vi "convertDATACluster.vi"(0 "Variable header":string[](array[string]), 5 "Alias":string[](array[string]), 7 "Array 6":bool[](array[boolean]), 9 "Data in":string[][](array[string]), 12 "variant in":variant) -> (2 "Array of VData":variant[](array[variant]), 3 "type":T5[](array[typedef]) format="%.0x", 4 "Array 2":u32[](array[numeric]), 6 "userID":string, 8 "Array":T5[](array[typedef]) format="%.0x", 10 "Array 3":u32[](array[numeric]), 13 "post time":u32, 14 "Array 4":u32[](array[numeric]), 15 "variant out":variant)   [LabVIEW 2011]
uses:
  <userlib>/_OpenG.lib/lvdata/lvdata.llb/Type Descriptor Enumeration__ogtk.ctl
  dataTypdef.ctl
  <vilib>/vision/Image Controls.llb/IMAQ Image.ctl
  ROIStartfromCam_typdef.ctl
  classicROI_typDef.ctl
  <userlib>/_OpenG.lib/array/array.llb/Sort 2D Array (I32)__ogtk.vi
  <vilib>/vision/NI_Vision_Development_Module.lvlib
panel:
  out "element Name":string[](array[string])
  out "index Array":i32[][](array[numeric])
  out "Sorted Array out":i32[][](array[numeric])
  out "clusterIndex (stop)":i32[](array[numeric])
  out "Array 5":variant[](array[variant])
  out "clusterIndex":i32[](array[numeric])
  out "Cluster Names":string[](array[string])
  out "data 3":T1
  in  "Cam2":T1
  out "VCluster 2":variant
  out "deleted portion":variant[](array[variant])
  out "Array 9":variant[](array[variant])
  out "VCluster":variant
  out "Names (Array)":string[](array[string])
  out "Array 8":bool[](array[boolean])
  out "Array 7":i32[](array[numeric])
  out "data 2":T2
  in  "data":T2
  out "transposed array":string[][](array[string])
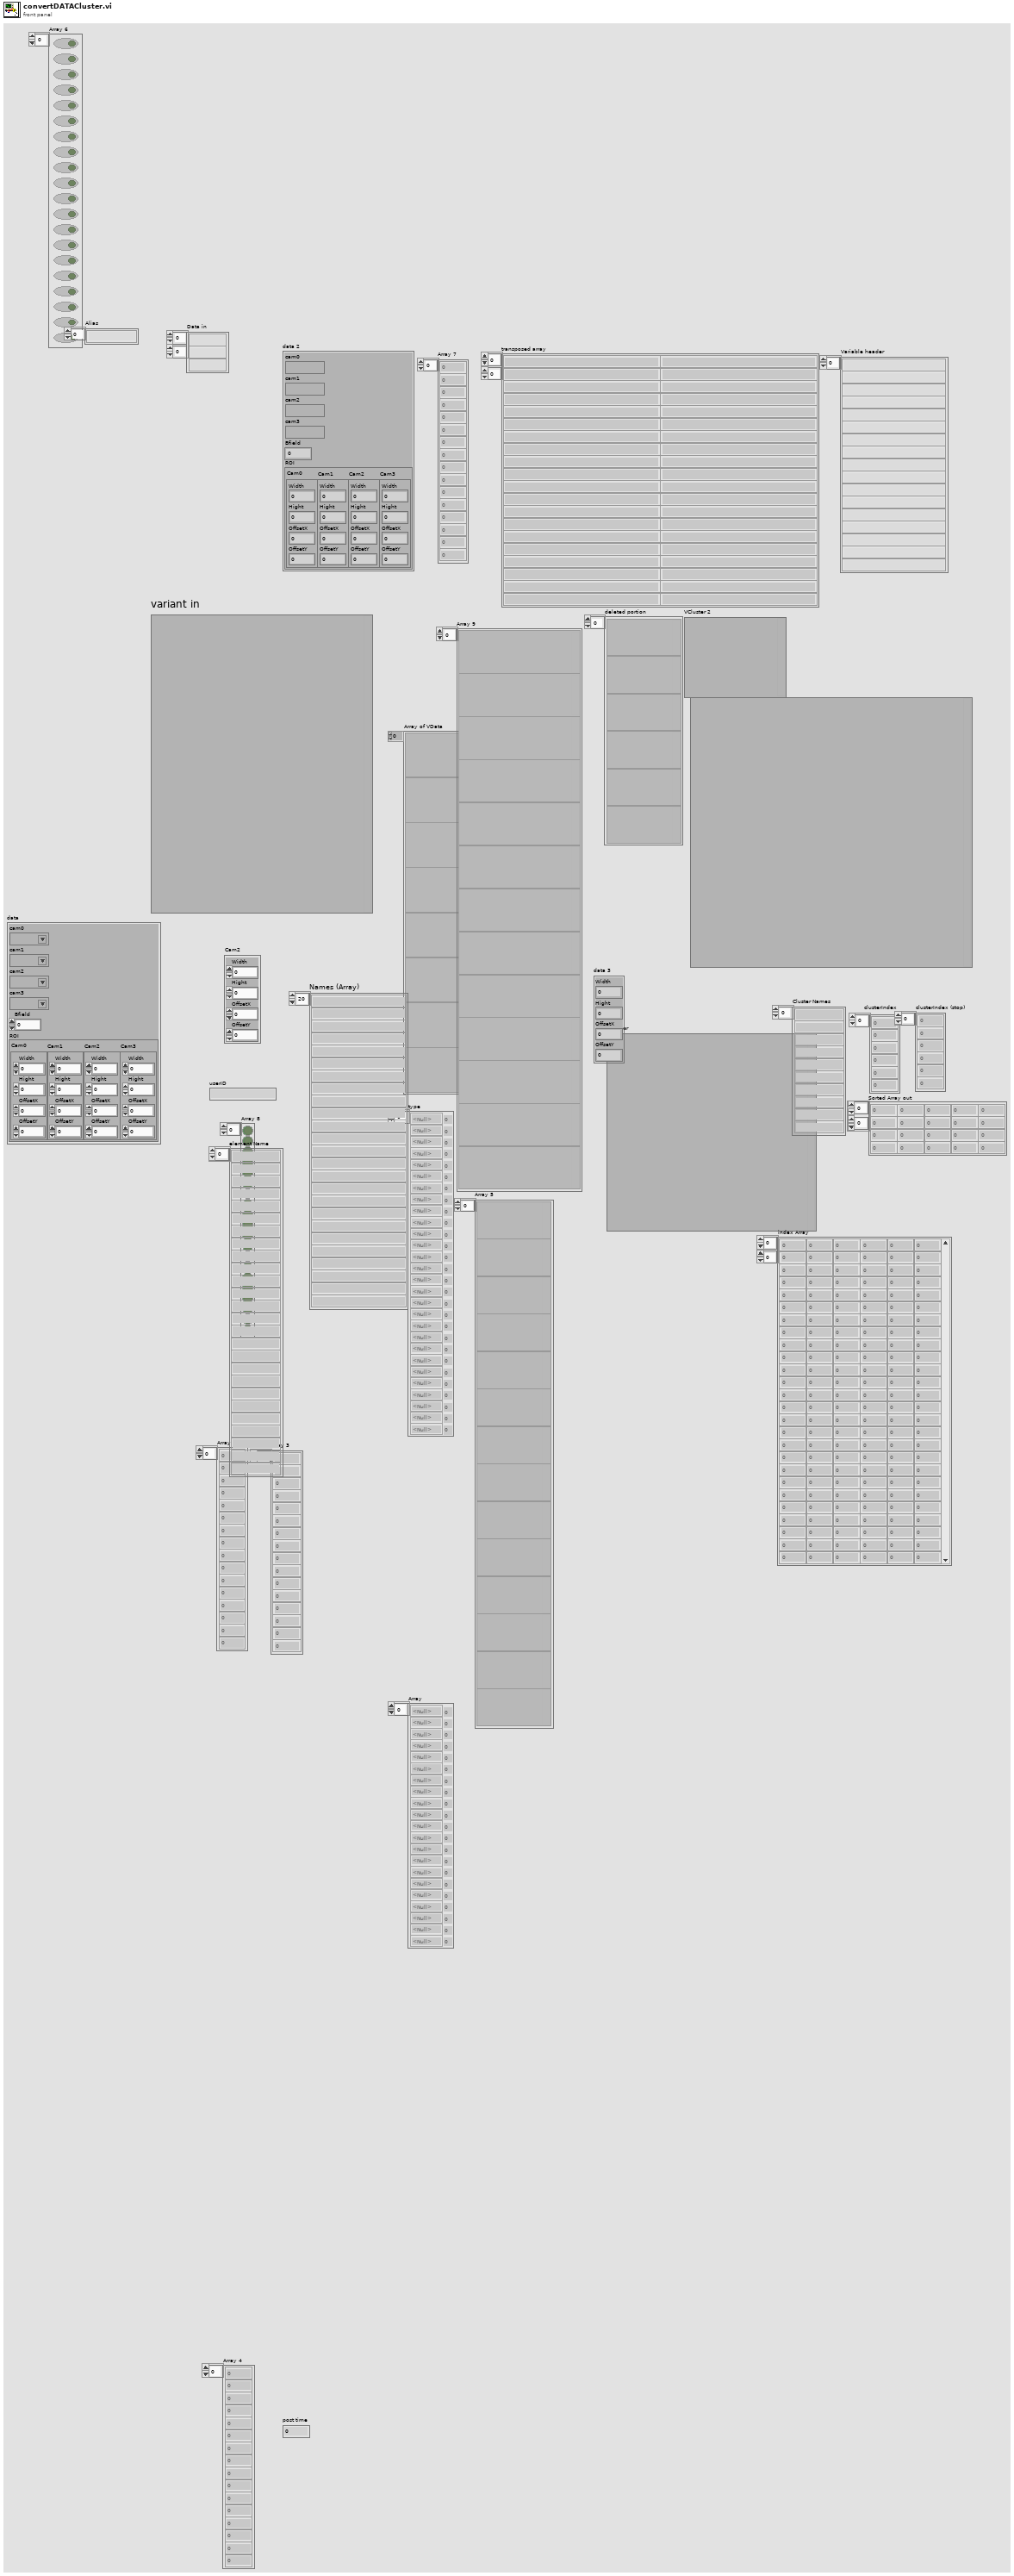
[diagram p1: front panel]
types:
  T1 = typedef "classicROI_typDef.ctl" = cluster{"Width":dbl, "Hight":dbl, "OffsetX":dbl, "OffsetY":dbl}
  T2 = typedef "dataTypdef.ctl" = cluster{"cam0":T3, "cam1":T3, "cam2":T3, "cam3":T3, "Bfield":dbl, "ROI":T4}
  T3 = typedef "IMAQ Image.ctl" = refnum<image>
  T4 = typedef "ROIStartfromCam_typdef.ctl" = cluster{"Cam0":T1, "Cam1":T1, "Cam2":T1, "Cam3":T1}
  T5 = typedef "Type Descriptor Enumeration__ogtk.ctl" = enum8{"<Null>", "I8", "I16", "I32", "I64", "U8", "U16", "U32", "U64", "SGL", "DBL", "EXT", "CSG", "CDB", "CXT", "0x0F", "0x10", "0x11", "0x12", "0x13", "0x14", "Enum U8", "Enum U16", "Enum U32", "Enum U64", "SGL PQ", "DBL PQ", "EXT PQ", "CSG PQ", "CDB PQ", "CXT PQ", "0x1F", "0x20", "Boolean", "0x22", "0x23", "0x24", "0x25", "0x26", "0x27", "0x28", "0x29", "0x2A", "0x2B", "0x2C", "0x2D", "0x2E", "0x2F", "String", "0x31", "Path", "Pict", "0x34", "0x35", "0x36", "DAQ", "0x38", "0x39", "0x3A", "0x3B", "0x3C", "0x3D", "0x3E", "0x3F", "Array", "0x41", "0x42", "0x43", "0x44", "0x45", "0x46", "0x47", "0x48", "0x49", "0x4A", "0x4B", "0x4C", "0x4D", "0x4E", "0x4F", "Cluster", "0x51", "0x52", "Variant", "Waveform", "0x55", "0x56", "0x57", "0x58", "0x59", "0x5A", "0x5B", "0x5C", "0x5D", "0x5E", "0x5F", "0x60", "0x61", "0x62", "0x63", "0x64", "0x65", "0x66", "0x67", "0x68", "0x69", "0x6A", "0x6B", "0x6C", "0x6D", "0x6E", "0x6F", "Refnum"}
  T6 = typedef "Image Type" = u32
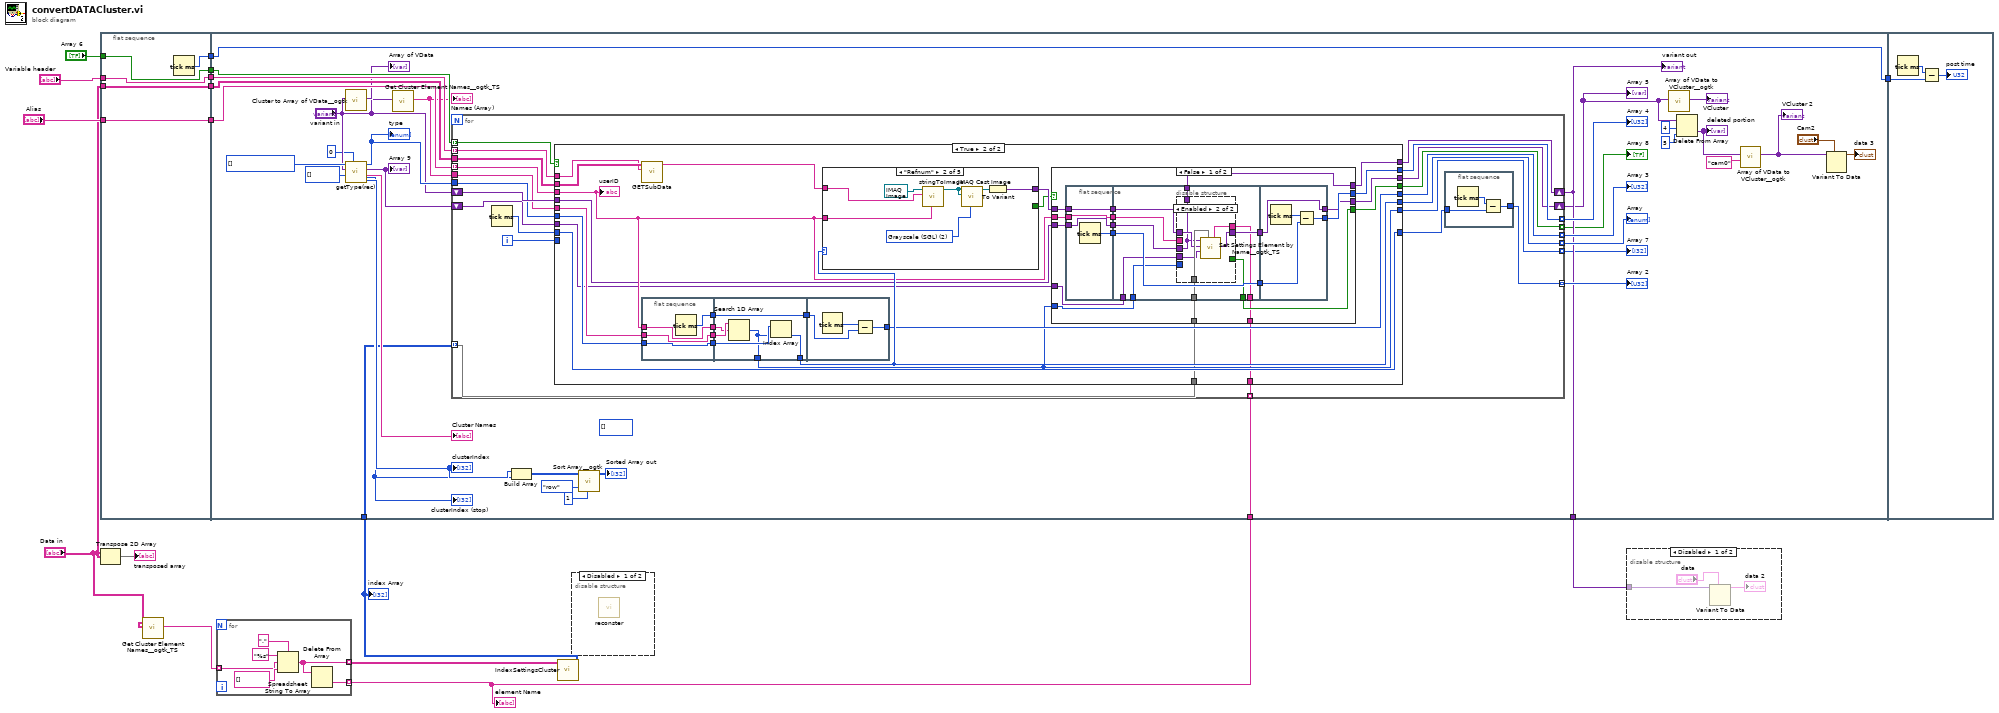
[diagram p0: block diagram]
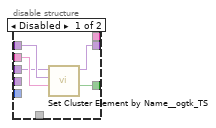
[diagram p5: hidden frame]
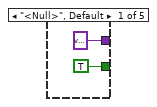
[diagram p7: hidden frame]
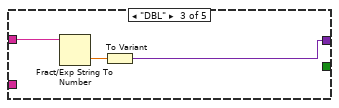
[diagram p8: hidden frame]
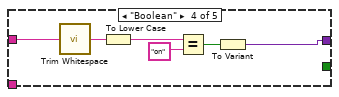
[diagram p9: hidden frame]
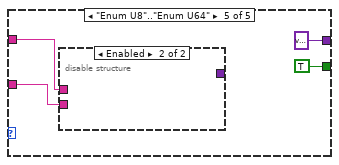
[diagram p10: hidden frame]
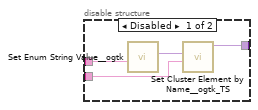
[diagram p11: hidden frame]
diagram:
  n1 = flat-sequence {
    tunnel: "Array 6" -> [w18]
    tunnel: "Alias" -> [w19]
    tunnel: "Data in" -> [w20]
    tunnel: "Variable header" -> [w21]
    tunnel: [w21] -> w16
    tunnel: [w20] -> w15
    tunnel: [w19] -> w14
    tunnel: [w18] -> w13
    tunnel: [w17] -> w12
    tunnel: w16 -> [w59]
    tunnel: w15 -> [w58]
    tunnel: w14 -> [w51]
    tunnel: w13 -> [w57]
    tunnel: w12 -> [w56]
    tunnel: [w56] -> w11
    tunnel: [w45] -> w6
    tunnel: w4 -> [w23]
    tunnel: w1 -> [w22]
    tunnel: w11 -> [w201]
    frame #0 {
      n2 = Tick Count (ms)() -> (millisecond timer value=w17:u32)
    }
    frame #1 {
      (unwired) i32[] [] ("clusterinex")
      w52 = T5[] [] items=["<Null>", "I8", "I16", "I32", "I64", "U8", "U16", "U32", "U64", "SGL", "DBL", "EXT", "CSG", "CDB", "CXT", "0x0F", "0x10", "0x11", "0x12", "0x13", "0x14", "Enum U8", "Enum U16", "Enum U32", "Enum U64", "SGL PQ", "DBL PQ", "EXT PQ", "CSG PQ", "CDB PQ", "CXT PQ", "0x1F", "0x20", "Boolean", "0x22", "0x23", "0x24", "0x25", "0x26", "0x27", "0x28", "0x29", "0x2A", "0x2B", "0x2C", "0x2D", "0x2E", "0x2F", "String", "0x31", "Path", "Pict", "0x34", "0x35", "0x36", "DAQ", "0x38", "0x39", "0x3A", "0x3B", "0x3C", "0x3D", "0x3E", "0x3F", "Array", "0x41", "0x42", "0x43", "0x44", "0x45", "0x46", "0x47", "0x48", "0x49", "0x4A", "0x4B", "0x4C", "0x4D", "0x4E", "0x4F", "Cluster", "0x51", "0x52", "Variant", "Waveform", "0x55", "0x56", "0x57", "0x58", "0x59", "0x5A", "0x5B", "0x5C", "0x5D", "0x5E", "0x5F", "0x60", "0x61", "0x62", "0x63", "0x64", "0x65", "0x66", "0x67", "0x68", "0x69", "0x6A", "0x6B", "0x6C", "0x6D", "0x6E", "0x6F", "Refnum"] ("type in")
      n3 = call <userlib>:"Cluster to Array of VData__ogtk.vi"("Cluster"="variant in") -> ("Array of VData"=→"Array of VData":variant[])  [unwired: 9 in, 1 out]
      n4 = call "getType(rec).vi"("index"=0, "clusterIndex (start)"=i32[] [], "variant in"="variant in", "type in"=w52) -> ("clusterIndex (start)"=w29:i32[], "Cluster Names"=→"Cluster Names":string[], "Array 2"=w42:variant[], "Array"=w49:T5[], "clusterIndex (stop)"=w28:i32[])  [unwired: 2 in, 1 out]
      "type" <- w49
      "Array 9" <- w42
      "clusterIndex" <- w29
      "clusterIndex (stop)" <- w28
      n5 = call "Get Cluster Element Names__ogtk_TS.vi"("Variant"="variant in") -> ("Names (Array)"=w47:string[])  [unwired: 9 in, 1 out]
      "Names (Array)" <- w47
      n6 = for {
        tunnel: w58 -> [w79]
        shift-right: [w80] -> w45
        shift-left: "variant in" -> [w77]
        tunnel: w59 -> [w78] mode=indexing
        tunnel: w51 -> [w76] mode=indexing
        tunnel: w57 -> [w75] mode=indexing
        tunnel: [w74] -> w55 mode=indexing
        tunnel: [w71] -> w54 mode=indexing
        tunnel: [w70] -> w53 mode=indexing
        tunnel: w49 -> [w68]
        tunnel: w47 -> [w67]
        tunnel: [w66] -> w46 mode=indexing
        tunnel: [w65] -> w44 mode=indexing
        tunnel: [w64] -> w43 mode=indexing
        shift-right: [w62] -> w31
        shift-left: w42 -> [w63]
        tunnel: w23 -> [w61] mode=indexing
        tunnel: w22 -> [w60] mode=indexing
        i -> [w69]
        n7 = Tick Count (ms)() -> (millisecond timer value=w73:u32)
        n8 = case shown="True" w75 {
          tunnel: [w86 w98] -> w80
          tunnel: w79 -> [_ w111]
          tunnel: w78 -> [_ w110]
          tunnel: w77 -> [w86 w92]
          tunnel: w76 -> [_ w96]
          tunnel: [_ w105] -> w74
          tunnel: w73 -> [w85 w108]
          tunnel: [w85 w108] -> w72
          tunnel: [_ w99] -> w70
          tunnel: w69 -> [_ _]
          tunnel: w68 -> [_ w106]
          tunnel: w67 -> [_ w107]
          tunnel: [_ w94] -> w66
          tunnel: [_ w89] -> w65
          tunnel: [_ w93] -> w64
          tunnel: w63 -> [w84 w91]
          tunnel: [w84 w90] -> w62
          tunnel: w61 -> [_ w88]
          tunnel: w60 -> [_ w87]
          frame False {
          }
          frame True {
            n9 = call "GETSubData.vi"("Variable Header"=w110, "Data out"=w111) -> ("delimiter (Tab)"=w109:string)  [unwired: 9 in]
            n10 = flat-sequence {
              tunnel: w106 -> [w162]
              tunnel: w96 -> [w163]
              tunnel: w107 -> [w164]
              tunnel: [w164] -> w104
              tunnel: [w163] -> w103
              tunnel: [w162] -> w102
              tunnel: [w161] -> w101
              tunnel: [w167] -> w105
              tunnel: w104 -> [w170]
              tunnel: w103 -> [w169]
              tunnel: w102 -> [w168]
              tunnel: w101 -> [w166]
              tunnel: [w166] -> w100
              tunnel: [w165] -> w89
              tunnel: w100 -> [w172]
              tunnel: [w171] -> w99
              frame #0 {
                n11 = Tick Count (ms)() -> (millisecond timer value=w161:u32)
              }
              frame #1 {
                n12 = Search 1D Array(1D array=w170, element=w169) -> (index of element=w165:i32)  [unwired: 1 in]
                n13 = Index Array(array=w168, index=w165) -> (element=w167:T5)
              }
              frame #2 {
                n14 = Tick Count (ms)() -> (millisecond timer value=w173:u32)
                n15 = Subtract(x=w173, y=w172) -> (x-y=w171:u32)
              }
            }
            n16 = case shown="\"Refnum\"" w105 {
              tunnel: w109 -> [_ w182 w185 w191 w195]
              tunnel: w96 -> [_ w176 _ _ w194]
              tunnel: [variant ("Variant") w177 w183 w186 variant ("Variant")] -> w97
              tunnel: [TRUE _ _ _ TRUE] -> w95
              frame "<Null>", Default {
              }
              frame "Refnum" {
                w180 = T6 2 items=["Grayscale (U8)", "Grayscale (I16)", "Grayscale (SGL)", "Complex (CSG)", "RGB (U32)", "HSL (U32)", "RGB (U64)", "Grayscale (U16)"] ("Image Type")
                n17 = call "stringToImage.vi"("label text (image name)"=w176, "data out"=w182, "Refnum in"=T3 refnum ("Image")) -> ("Refnum out"=w181:T3)  [unwired: 5 in, 3 out]
                n18 = call "IMAQ Cast Image"("Image Type"=w180, "Image Dst"=w181, "Image Src"=w181) -> ("Image Dst Out"=w178:T3)  [unwired: 7 in, 1 out]
                n19 = To Variant(anything=w178) -> (Variant=w177:variant)
              }
              frame "DBL" {
                n20 = Fract/Exp String To Number(string=w185) -> (number=w184:dbl)  [unwired: 3 in, 1 out]
                n21 = To Variant(anything=w184) -> (Variant=w183:variant)
              }
              frame "Boolean" {
                n22 = call <vilib>:"Trim Whitespace.vi"("string"=w191) -> ("trimmed string"=w190:string)  [unwired: 1 in]
                n23 = To Lower Case(string=w190) -> (all lower case string=w189:string)
                n24 = Equal?(x=w189, y="on" ("x")) -> (x = y?=w187:bool)
                n25 = To Variant(anything=w187) -> (Variant=w186:variant)
              }
              frame "Enum U8".."Enum U64" {
                n26 = disable-structure shown="Enabled" {
                  disable-tunnel: w195 -> [w199 _]
                  disable-tunnel: w194 -> [w198 _]
                  disable-tunnel: [w196 _] -> _
                  frame Disabled {
                    n27 = call <userlib>:"Set Enum String Value__ogtk.vi"("String Value"=w199) -> ("Enum"=w197:variant)  [unwired: 9 in, 1 out]
                    n28 = call "Set Cluster Element by Name__ogtk_TS.vi"("Element Name (\"\": New Element Data Name)"=w198, "New Element Value"=w197) -> ("VCluster out"=w196:variant)  [unwired: 7 in, 2 out]
                  }
                  frame Enabled {
                  }
                }
              }
            }
            n29 = case shown="False" w95 {
              tunnel: w92 -> [w128 w160]
              tunnel: [w113 w160] -> w98
              tunnel: w97 -> [w127 _]
              tunnel: w96 -> [w126 _]
              tunnel: [w120 _] -> w94
              tunnel: [w119 _] -> w93
              tunnel: w91 -> [w117 w159]
              tunnel: [w114 w159] -> w90
              tunnel: w89 -> [w116 _]
              tunnel: w88 -> [w115 _]
              tunnel: w87 -> [w112 _]
              frame False {
                n30 = flat-sequence {
                  tunnel: w126 -> [w130]
                  tunnel: w127 -> [w131]
                  tunnel: w128 -> [w132]
                  tunnel: [w132] -> w125
                  tunnel: [w131] -> w124
                  tunnel: [w130] -> w123
                  tunnel: [w129] -> w122
                  tunnel: w125 -> [w138]
                  tunnel: w124 -> [w140]
                  tunnel: w123 -> [w141]
                  tunnel: w122 -> [w143]
                  tunnel: [w143] -> w121
                  tunnel: [w142] -> w119
                  tunnel: [w139] -> w118
                  tunnel: w117 -> [w137]
                  tunnel: w116 -> [w136]
                  tunnel: w115 -> [w135]
                  tunnel: [w134] -> w113
                  tunnel: w112 -> [w133]
                  tunnel: w121 -> [w157]
                  tunnel: [w156] -> w120
                  tunnel: w118 -> [w155]
                  tunnel: [w155] -> w114
                  frame #0 {
                    n31 = Tick Count (ms)() -> (millisecond timer value=w129:u32)
                  }
                  frame #1 {
                    n32 = disable-structure shown="Enabled" {
                      disable-tunnel: [w148 _] -> w142
                      disable-tunnel: w141 -> [w147 _]
                      disable-tunnel: w140 -> [w146 w153]
                      disable-tunnel: [w145 w151] -> w139
                      disable-tunnel: w138 -> [w144 w150]
                      disable-tunnel: w137 -> [_ w152]
                      disable-tunnel: w136 -> [_ _]
                      disable-tunnel: w135 -> [_ w154]
                      disable-tunnel: [_ w150] -> w134
                      disable-tunnel: w133 -> [_ w149]
                      frame Disabled {
                        n33 = call "Set Cluster Element by Name__ogtk_TS.vi"("Element Name (\"\": New Element Data Name)"=w147, "New Element Value"=w146, "Cluster"=w144) -> ("found?"=w148:bool, "VCluster out"=w145:variant)  [unwired: 6 in, 1 out]
                      }
                      frame Enabled {
                        n34 = call "Set Settings Element by Name__ogtk_TS.vi"("element Name"=w149, "index Array"=w154, "Settings VData"=w152, "New Element Value"=w153, "Cluster"=w150) -> ("Settings VData out"=w151:variant[])  [unwired: 5 in, 1 out]
                      }
                    }
                  }
                  frame #2 {
                    n35 = Tick Count (ms)() -> (millisecond timer value=w158:u32)
                    n36 = Subtract(x=w158, y=w157) -> (x-y=w156:u32)
                  }
                }
              }
              frame True {
              }
            }
            "userID" <- w96
          }
        }
        n37 = flat-sequence {
          tunnel: w72 -> [w82]
          tunnel: [w81] -> w71
          frame #0 {
            n38 = Tick Count (ms)() -> (millisecond timer value=w83:u32)
            n39 = Subtract(x=w83, y=w82) -> (x-y=w81:u32)
          }
        }
      }
      "variant out" <- w45
      "Array" <- w55
      "Array 2" <- w54
      "Array 3" <- w53
      "Array 4" <- w46
      "Array 7" <- w44
      "Array 8" <- w43
      "Array 5" <- w31
      n40 = Build Array(w29, w28) -> (w27:i32[][])
      n41 = call-poly <userlib>:"Sort Array__ogtk.vi"("Column/Row to Sort By"=u32 1, "Sort By in"=enum16{"row", "column"}."row", "Array in"=w27) -> ("Sorted Array out"=→"Sorted Array out":i32[][])  [unwired: 5 in, 3 out]
      n42 = call <userlib>:"Array of VData to VCluster__ogtk.vi"("Array"=w31) -> ("VCluster"=→"VCluster":variant)  [unwired: 9 in, 1 out]
      n43 = Delete From Array(array=w31, length=4, index=5) -> (deleted portion=w38:variant[])  [unwired: 1 out]
      "deleted portion" <- w38
      n44 = call <userlib>:"Array of VData to VCluster__ogtk.vi"("Cluster Name"="cam0", "Array"=w38) -> ("VCluster"=w36:variant)  [unwired: 8 in, 1 out]
      "VCluster 2" <- w36
      n45 = Variant To Data(type="Cam2", Variant=w36) -> (data=→"data 3":T1)  [unwired: 1 in, 1 out]
    }
    frame #2 {
      n46 = Tick Count (ms)() -> (millisecond timer value=w202:u32)
      n47 = Subtract(x=w202, y=w201) -> (x-y=→"post time":u32)
    }
  }
  n48 = Transpose 2D Array(2D array="Data in") -> (transposed array=→"transposed array":string[][])
  n49 = call "Get Cluster Element Names__ogtk_TS.vi"("Variant"="Data in") -> ("Names (Array)"=w2:string[])  [unwired: 9 in, 1 out]
  n50 = for {
    tunnel: w2 -> [w205] mode=indexing
    tunnel: [w204] -> w5 mode=indexing
    tunnel: [w203] -> w1 mode=indexing
    n51 = Spreadsheet String To Array(delimiter (Tab)=".", format string="%s", spreadsheet string=w205, array type (2D Dbl)=string[] []) -> (array=w204:string[])
    n52 = Delete From Array(array=w204) -> (deleted portion=w203:string)  [unwired: 2 in, 1 out]
  }
  "element Name" <- w1
  n53 = call "IndexSettingsCluster.vi"("Names Array"=w5) -> ("index Array"=w4:i32[][])  [unwired: 10 in]
  "index Array" <- w4
  n54 = disable-structure shown="Disabled" {
    frame Disabled {
      n55 = call "reconster.vi"() -> ()  [unwired: 12 in]
    }
    frame Enabled {
    }
  }
  n56 = disable-structure shown="Disabled" {
    disable-tunnel: w6 -> [w211 _]
    frame Disabled {
      n57 = Variant To Data(type="data", Variant=w211) -> (data=→"data 2":T2)  [unwired: 1 in, 1 out]
    }
    frame Enabled {
    }
  }
